vi "Set Config Digitals.vi"(0 "connection ID":refnum<k16>, 1 "address":u32, 2 "port":u16, 5 "Digital Number":u16, 7 "Digital Mode":T1=73 items=["Output"=79, "Input_Pullup"=80, "Input"=73], 9 "timeout ms (1000)":i32=1000, 11 "error in (no error)":errorcluster, 12 "mask":u16) -> (4 "connection ID out":refnum<k16>, 6 "received data":string, 15 "error out":errorcluster)   [LabVIEW 2016, in "instr.lvlib"]
doc: "Sets given digital io to given digital mode."
uses:
  instr.lvlib
  Digital Mode.ctl
panel:
  out "Send String":string
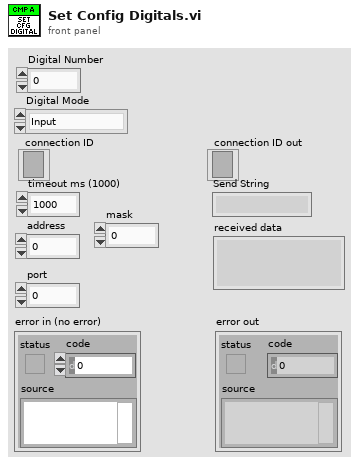
[diagram p1: front panel]
types:
  T1 = typedef "instr.lvlib/Digital Mode.ctl" = u16
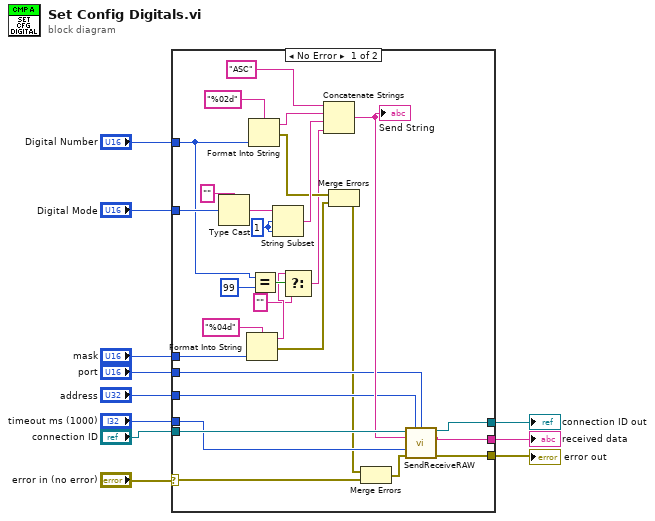
[diagram p0: block diagram]
diagram:
  n1 = case shown="No Error" "error in (no error)" {
    selector: "error in (no error)" -> [w38 w42]
    tunnel: [w36 w42] -> w11
    tunnel: [w35 _] -> w9
    tunnel: "timeout ms (1000)" -> [w31 _]
    tunnel: "connection ID" -> [w33 w41]
    tunnel: [w34 w41] -> w6
    tunnel: "Digital Number" -> [w12 _]
    tunnel: "address" -> [w29 _]
    tunnel: "port" -> [w28 _]
    tunnel: "Digital Mode" -> [w27 _]
    tunnel: "mask" -> [w13 _]
    frame No Error {
      w24 = 1 ("offset (0)")
      n2 = Type Cast(type="", x=w27) -> (*(type *) &x=w25:string)
      n3 = Format Into String(format string="%04d", w13) -> (resulting string=w19:string, error out=w16:errorcluster)  [unwired: 2 in]
      n4 = Format Into String(format string="%02d", w12) -> (resulting string=w37:string, error out=w17:errorcluster)  [unwired: 2 in]
      n5 = Equal?(x=w12, y=u16 99) -> (x = y?=w20:bool)
      n6 = String Subset(string=w25, offset (0)=w24, length (rest)=w24) -> (substring=w23:string)
      n7 = Select(t=w19, s=w20, f="") -> (s? t:f=w14:string)
      n8 = Concatenate Strings("ASC" ("data in"), w37, w23, w14) -> (w30:string)
      "Send String" <- w30
      n9 = Merge Errors(w17, w16) -> (w15:errorcluster)
      n10 = Merge Errors(w15, w38) -> (w32:errorcluster)
      n11 = call "SendReceiveRAW.vi"("connection ID"=w33, "address"=w29, "port"=w28, "RAW data in"=w30, "timeout ms (1000)"=w31, "error in (no error)"=w32) -> ("connection ID out"=w34:refnum<k16>, "received data"=w35:string, "error out"=w36:errorcluster)  [unwired: 7 in]
    }
    frame Error {
    }
  }
  "error out" <- w11
  "received data" <- w9
  "connection ID out" <- w6
